vi "Trigger Start Event.vi"(8 "error in (no error)":errorcluster) -> (0 "error out":errorcluster)   [LabVIEW 2024, in "View.lvlib"]
uses:
  View.lvlib
  Type Defs/Start Event Args--cluster.ctl
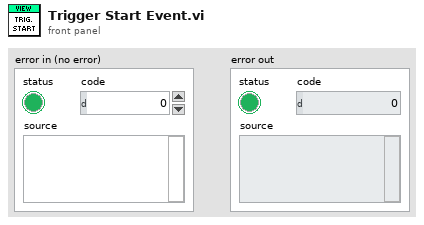
[diagram p1: front panel]
types:
  T1 = typedef "View.lvlib/Start Event Args--cluster.ctl" = cluster{"None":bool}
  T2 = cluster{"Start Event":refnum<user-event>, "Pause Event":refnum<user-event>, "Stop Event":refnum<user-event>}
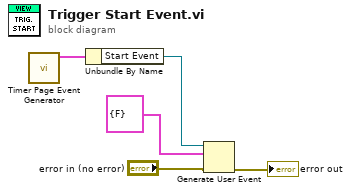
[diagram p0: block diagram]
diagram:
  n1 = call "Timer Page Event Generator.vi"() -> ("Timer Events"=w5:T2)  [unwired: 10 in, 1 out]
  n2 = Unbundle By Name(w5) -> ("Start Event"=w4:refnum<user-event>)
  n3 = Generate User Event(user event=w4, event data cluster=T1 {"None"=FALSE} ("Start Event Input"), error in="error in (no error)") -> (error out=→"error out":errorcluster)  [unwired: 1 in, 1 out]
